vi "Control System Definition API Example.vi"(10 "Control Addon Config Datalog Path":path, 11 "Existing SysDef Path":path) -> (0 "error out":errorcluster)   [LabVIEW 2019]
uses:
  NationalInstruments.VeriStand.SystemDefinitionAPI
  Control System Definition API.lvlib
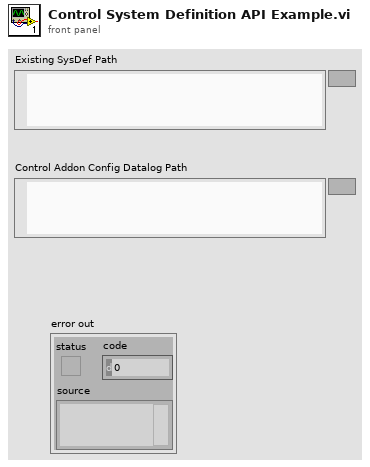
[diagram p1: front panel]
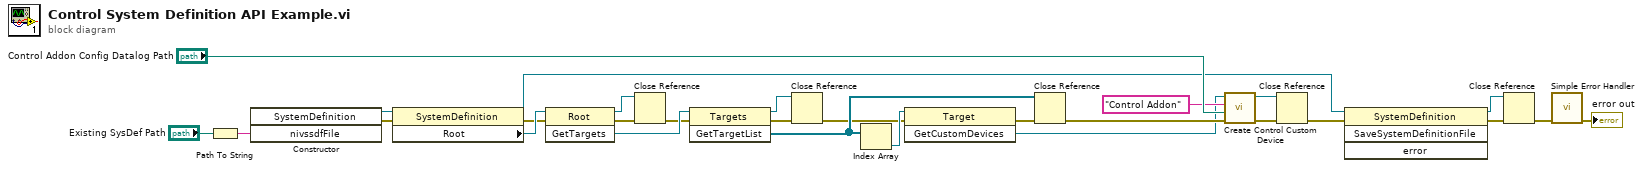
[diagram p0: block diagram]
diagram:
  n1 = Path To String(path="Existing SysDef Path") -> (string=w1:string)
  n2 = constructor class="SystemDefinition"("nivssdfFile"=w1) -> (reference out=w28:refnum<k24>, error out=w24:errorcluster)  [unwired: 3 in, 2 out]
  n3 = property class="SystemDefinition"(reference=w28, error in=w24) -> (reference out=w2:refnum<k24>, error out=w23:errorcluster, "Root"=w27:refnum<k24>)
  n4 = invoke class="Root" method="GetTargets"(reference=w27, error in=w23) -> (reference out=w9:refnum<k24>, error out=w11:errorcluster, "GetTargets"=w26:refnum<k24>)  [unwired: 1 in]
  n5 = Close Reference(reference=w9, error in (no error)=w11) -> (error out=w10:errorcluster)
  n6 = invoke class="Targets" method="GetTargetList"(reference=w26, error in=w10) -> (reference out=w12:refnum<k24>, error out=w14:errorcluster, "GetTargetList"=w15:refnum<k24>[])  [unwired: 1 in]
  n7 = Close Reference(reference=w12, error in (no error)=w14) -> (error out=w13:errorcluster)
  n8 = Index Array(array=w15) -> (element=w25:refnum<k24>)  [unwired: 1 in]
  n9 = invoke class="Target" method="GetCustomDevices"(reference=w25, error in=w13) -> (error out=w17:errorcluster, "GetCustomDevices"=w5:refnum<k24>)  [unwired: 1 in, 1 out]
  n10 = Close Reference(reference=w15, error in (no error)=w17) -> (error out=w16:errorcluster)
  n11 = call "Create Control Custom Device.vi"("error in (no error)"=w16, "CD Config Path (.dat)"="Control Addon Config Datalog Path", "Name"="Control Addon", "Custom Devices Ref"=w5) -> ("error out"=w4:errorcluster, "Custom Devices Ref"=w18:refnum<k24>)  [unwired: 6 in]
  n12 = Close Reference(reference=w18, error in (no error)=w4) -> (error out=w19:errorcluster)
  n13 = invoke class="SystemDefinition" method="SaveSystemDefinitionFile"(reference=w2, error in=w19) -> (reference out=w20:refnum<k24>, error out=w21:errorcluster)  [unwired: 2 in, 2 out]
  n14 = Close Reference(reference=w20, error in (no error)=w21) -> (error out=w8:errorcluster)
  n15 = call <vilib>:"Simple Error Handler.vi"("error in (no error)"=w8) -> ("error out"=→"error out":errorcluster)  [unwired: 4 in, 4 out]
